vi "elapsed_sec.vi"(8 "reset2":i32, 11 "reset":i32) -> (3 "params2":i32)   [LabVIEW 2015]
uses:
  BERTTA.dll
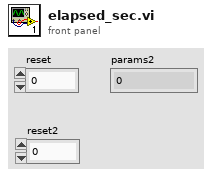
[diagram p1: front panel]
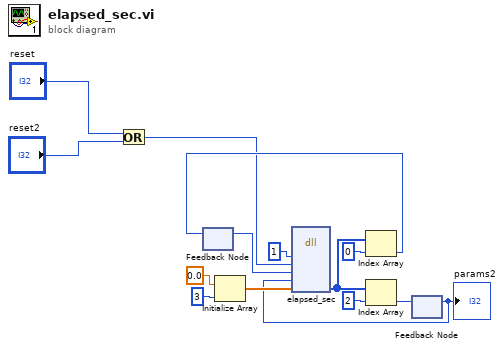
[diagram p0: block diagram]
diagram:
  n1 = Or(x="reset", y="reset2") -> (x .or. y?=w1:i32)
  n2 = feedback #1() -> (w7:i32)  [unwired: 1 in]
  n3 = Initialize Array(0.0 ("element"), 3 ("dimension size")) -> (w11:dbl[])
  n4 = feedback #2() -> (w5:i32)  [unwired: 1 in]
  "params2" <- w5
  n5 = dll-call lib="C:/Users/shresplab/OneDrive - Kemira Oyj/Documents/Visual Studio 2017/Projects/Bertta/BERTTA/x64/Debug/BERTTA.dll" fn="elapsed_sec"("enable"=1, "reset"=w1, "last_time"=w7, "elapsed_last"=w5, "params"=w11) -> ("params"=w9:i32[])  [unwired: 8 in, 2 out]
  n6 = Index Array(array=w9, index=0) -> (element=w8:i32)
  n7 = feedback-in #1(w8) -> ()
  n8 = Index Array(array=w9, index=2) -> (element=w6:i32)
  n9 = feedback-in #2(w6) -> ()
